vi "Test Model API.vi"() -> ()   [LabVIEW 2019]
doc: "Model API Tester."
uses:
  Model.lvlib
panel:
  in  "Show Block Diagram":bool
  in  "Stop Module":bool
  in  "Start Module":bool
  in  "Hide Module Panel":bool
  in  "Show Module Panel":bool
  out "Status":string
  out "Module Running?":bool
  # "This VI tests the API for the Module."
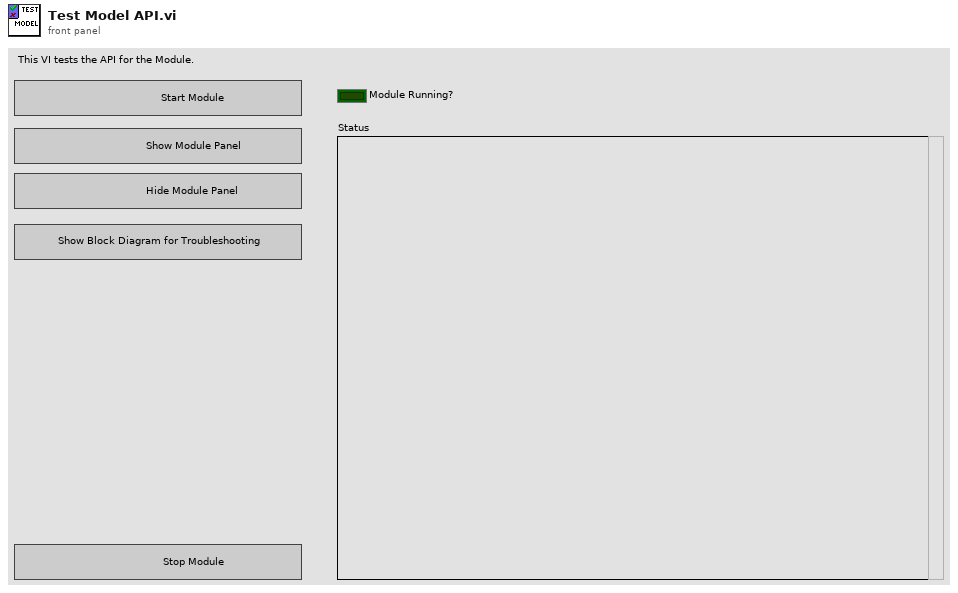
[diagram p1: front panel]
types:
  T1 = typedef "Model.lvlib/Broadcast Events--cluster.ctl" = cluster{"Module Did Init":refnum<user-event>, "Status Updated":refnum<user-event>, "Error Reported":refnum<user-event>, "Module Did Stop":refnum<user-event>, "Update Module Execution Status":refnum<user-event>}
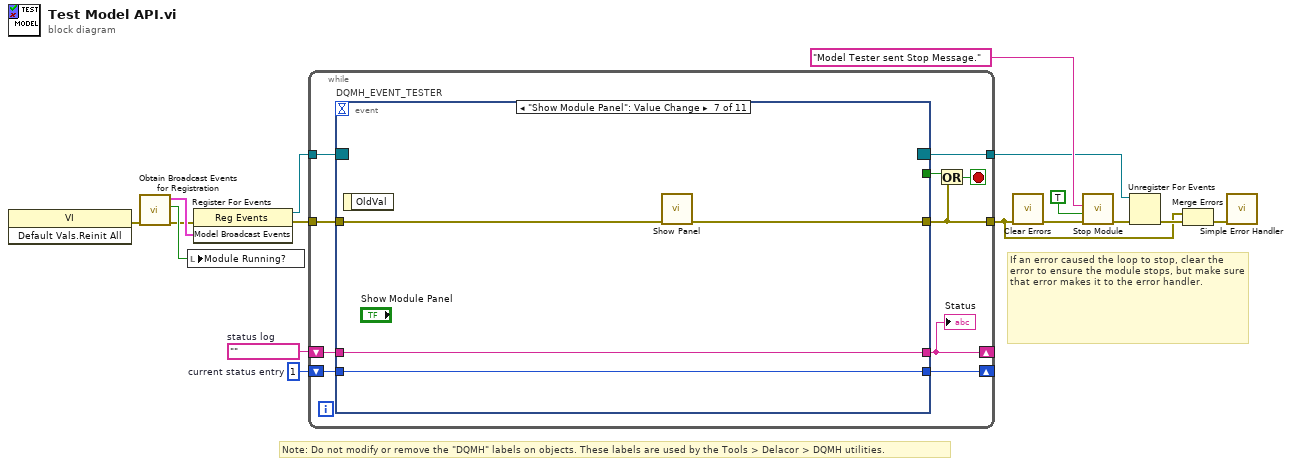
[diagram p0: block diagram]
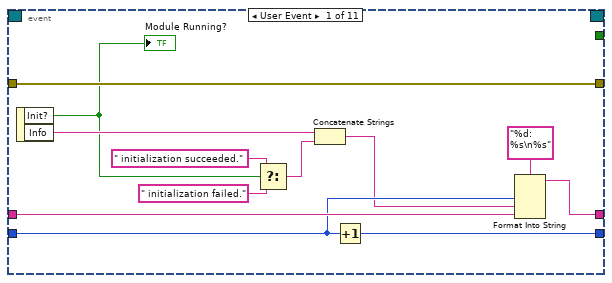
[diagram p2: hidden frame]
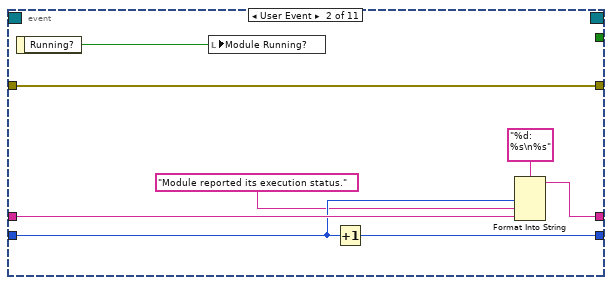
[diagram p3: hidden frame]
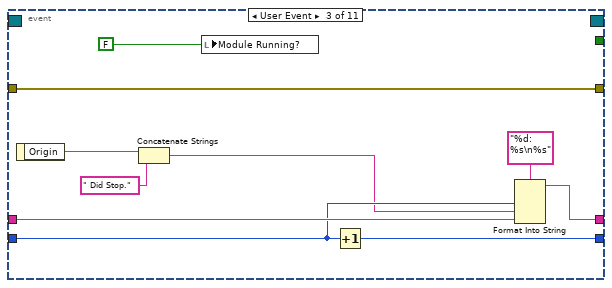
[diagram p4: hidden frame]
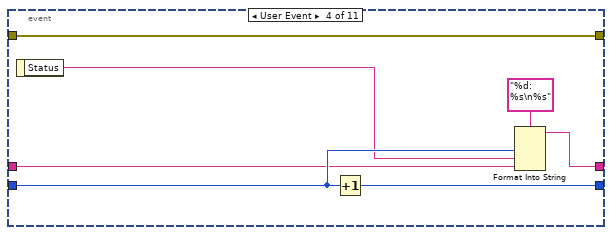
[diagram p5: hidden frame]
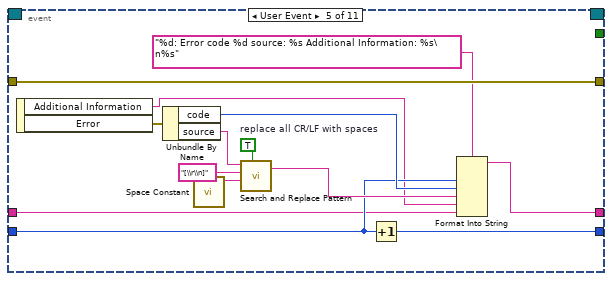
[diagram p6: hidden frame]
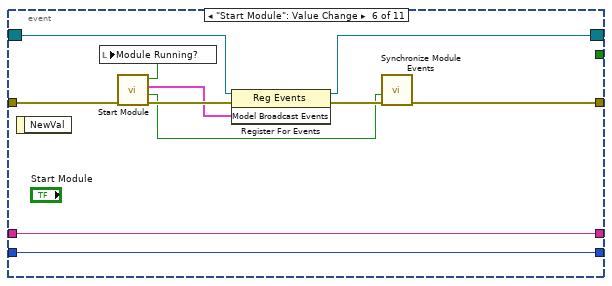
[diagram p7: hidden frame]
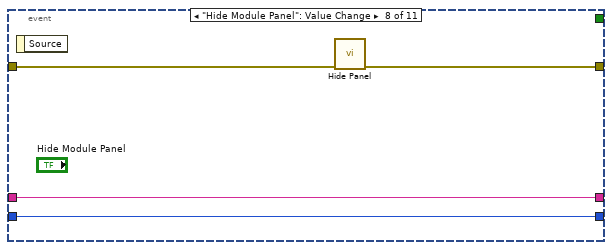
[diagram p8: hidden frame]
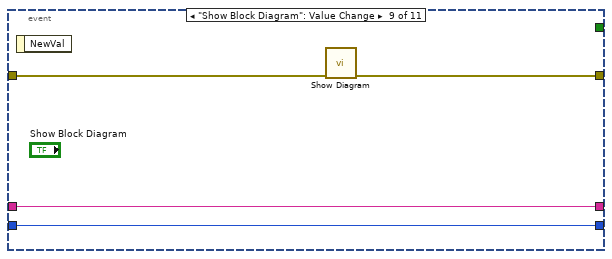
[diagram p9: hidden frame]
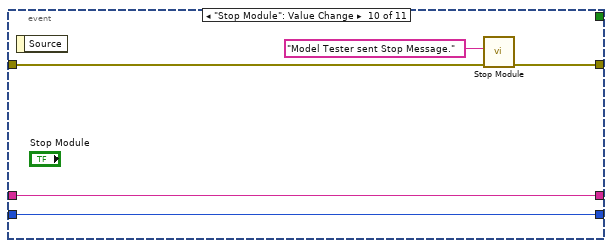
[diagram p10: hidden frame]
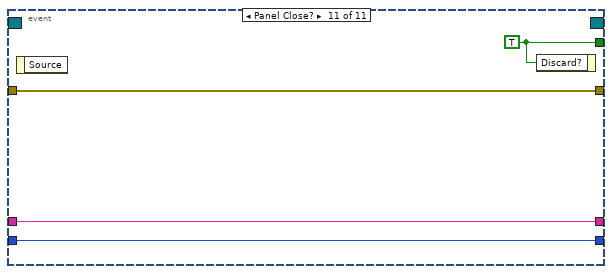
[diagram p11: hidden frame]
diagram:
  w12 = 1  # current status entry
  w13 = ""  # status log
  # "If an error caused the loop to stop, clear the error to ensure the module stops, but make sure that error makes it to the error handler."
  # "Note: Do not modify or remove the \"DQMH\" labels on objects. These labels are used by the Tools > Delacor > DQMH utilities."
  n1 = invoke class="VI" method="Default Vals.Reinit All"() -> (error out=w2:errorcluster)  [unwired: 3 in, 2 out]
  n2 = call "Obtain Broadcast Events for Registration.vi"("error in (no error)"=w2) -> ("error out"=w1:errorcluster, "Already running?"=w3:bool, "Model Broadcast Events"=w10:T1)  [unwired: 8 in]
  n3 = local write "Module Running?"(w3) -> ()
  n4 = register-events(error in=w1, w10) -> (reference out=w9:refnum<event-registration>, error out=w11:errorcluster)  [unwired: 1 in]
  n5 = while {
    tunnel: w9 -> [w26]
    tunnel: [w17] -> w4
    shift-right: [w21] -> _
    shift-left: w13 -> [w23]
    shift-right: [w22] -> _
    shift-left: w12 -> [w24]
    tunnel: w11 -> [w19]
    tunnel: [w18] -> w8
    stop <- w20 stop-if-true
    n6 = event "DQMH_EVENT_TESTER" shown="[6] \"Show Module Panel\": Value Change" {
      selector: w26 -> [_ _ _ _ _ w82 _ _ _ _ _]
      dyn-events: [_ _ _ _ _ w81 _ _ _ _ _] -> w18
      timeout: _ -> [_ _ _ _ _ _ _ _ _ _ _]
      tunnel: [_ _ _ _ _ _ _ _ _ _ w109] -> w25
      tunnel: [w38 w40 w47 w57 w77 w80 w92 w96 w97 w103 w106] -> w17
      tunnel: w24 -> [w35 w44 w54 w60 w67 w85 w90 w94 w98 w104 w107]
      tunnel: w23 -> [w36 w45 w55 w59 w65 w86 w91 w95 w99 w105 w108]
      tunnel: [w33 w42 w52 w61 w68 w86 w91 w95 w99 w105 w108] -> w21
      tunnel: [w34 w43 w53 w63 w66 w85 w90 w94 w98 w104 w107] -> w22
      tunnel: w19 -> [w38 w40 w47 w57 w77 w79 w89 w93 w100 w101 w106]
      event User Event {
        n7 = event-data() -> ("Init?"=w30:bool, "Info"=w32:string)  [unwired: 1 in]
        "Module Running?" <- w30
        n8 = Select(t=" initialization succeeded.", s=w30, f=" initialization failed.") -> (s? t:f=w27:string)
        n9 = Concatenate Strings(w32, w27) -> (w31:string)
        n10 = Increment(x=w35) -> (x+1=w34:i32)
        n11 = Format Into String(format string="%d: %s\n%s", w35, w31, w36) -> (resulting string=w33:string)  [unwired: 2 in, 1 out]
      }
      event User Event {
        n12 = event-data() -> ("Running?"=w39:bool)  [unwired: 1 in]
        n13 = local write "Module Running?"(w39) -> ()
        n14 = Increment(x=w44) -> (x+1=w43:i32)
        n15 = Format Into String(format string="%d: %s\n%s", w44, "Module reported its execution status.", w45) -> (resulting string=w42:string)  [unwired: 2 in, 1 out]
      }
      event User Event {
        n16 = event-data() -> ("Origin"=w51:string)  [unwired: 1 in]
        n17 = Concatenate Strings(w51, " Did Stop.") -> (w50:string)
        n18 = local write "Module Running?"(FALSE ("Module Did Init?")) -> ()
        n19 = Increment(x=w54) -> (x+1=w53:i32)
        n20 = Format Into String(format string="%d: %s\n%s", w54, w50, w55) -> (resulting string=w52:string)  [unwired: 2 in, 1 out]
      }
      event User Event {
        n21 = event-data() -> ("Status"=w58:string)  [unwired: 1 in]
        n22 = Increment(x=w60) -> (x+1=w63:i32)
        n23 = Format Into String(format string="%d: %s\n%s", w60, w58, w59) -> (resulting string=w61:string)  [unwired: 2 in, 1 out]
      }
      event User Event {
        w73 = TRUE  # replace all CR/LF with spaces
        n24 = event-data() -> ("Additional Information"=w64:string, "Error"=w69:errorcluster)  [unwired: 1 in]
        n25 = Unbundle By Name(w69) -> ("code"=w70:i32, "source"=w71:string)
        n26 = call <vilib>:"Space Constant.vi"() -> ("String"=w74:string)
        n27 = call <vilib>:"Search and Replace Pattern.vi"("string"=w71, "regular expression (\"\")"="[\\r\\n]" ("regular expression (\"\")"), "replace string (\"\")"=w74, "replace all? (F)"=w73) -> ("result string"=w72:string)  [unwired: 1 in, 1 out]
        n28 = Increment(x=w67) -> (x+1=w66:i32)
        n29 = Format Into String(format string="%d: Error code %d source: %s Additional Information: %s\n%s", w67, w70, w72, w64, w65) -> (resulting string=w68:string)  [unwired: 2 in, 1 out]
      }
      event "Start Module": Value Change {
        n30 = event-data() -> ()  [unwired: 1 in, 1 out]
        n31 = call "Start Module.vi"("error in (no error)"=w79) -> ("error out"=w87:errorcluster, "Wait for Event Sync?"=w84:bool, "Model Broadcast Events"=w83:T1, "Module Was Already Running?"=w78:bool)  [unwired: 7 in]
        n32 = local write "Module Running?"(w78) -> ()
        n33 = register-events(reference=w82, error in=w87, w83) -> (reference out=w81:refnum<event-registration>, error out=w88:errorcluster)
        n34 = call "Synchronize Module Events.vi"("error in (no error)"=w88, "Wait for Event Sync?"=w84) -> ("error out"=w80:errorcluster)  [unwired: 9 in]
      }
      event "Show Module Panel": Value Change {
        n35 = event-data() -> ()  [unwired: 1 in, 1 out]
        n36 = call "Show Panel.vi"("error in (no error)"=w89) -> ("error out"=w92:errorcluster)  [unwired: 10 in]
      }
      event "Hide Module Panel": Value Change {
        n37 = event-data() -> ()  [unwired: 1 in, 1 out]
        n38 = call "Hide Panel.vi"("error in (no error)"=w93) -> ("error out"=w96:errorcluster)  [unwired: 10 in]
      }
      event "Show Block Diagram": Value Change {
        n39 = event-data() -> ()  [unwired: 1 in, 1 out]
        n40 = call "Show Diagram.vi"("error in (no error)"=w100) -> ("error out"=w97:errorcluster)  [unwired: 10 in]
      }
      event "Stop Module": Value Change {
        n41 = event-data() -> ()  [unwired: 1 in, 1 out]
        n42 = call "Stop Module.vi"("error in (no error)"=w101, "Origin"="Model Tester sent Stop Message.") -> ("error out"=w103:errorcluster)  [unwired: 9 in]
      }
      event Panel Close? {
        w109 = TRUE ("Discard?")
        n43 = event-data() -> ()  [unwired: 1 in, 1 out]
        n44 = event-data("Discard?"=w109) -> ()  [unwired: 1 in, 1 out]
      }
    }
    "Status" <- w21
    n45 = Or(x=w25, y=w17) -> (x .or. y?=w20:bool)
  }
  n46 = call <vilib>:"Clear Errors.vi"("error in (no error)"=w4) -> ("error out"=w6:errorcluster)  [unwired: 5 in, 1 out]
  n47 = call "Stop Module.vi"("error in (no error)"=w6, "Wait for Module to Stop? (F)"=TRUE ("Wait for Module to stop?"), "Origin"="Model Tester sent Stop Message.") -> ("error out"=w15:errorcluster)  [unwired: 8 in]
  n48 = Unregister For Events(event registration refnum=w8, error in=w15) -> (error out=w16:errorcluster)
  n49 = Merge Errors(w4, w16) -> (w5:errorcluster)
  n50 = call <vilib>:"Simple Error Handler.vi"("error in (no error)"=w5) -> ()  [unwired: 4 in, 5 out]
